vi "Add test result.vi"(10 "Test Result":T1, 11 "LUnit Test Case In":refnum<class "LUnit Test Case.lvclass">) -> (3 "LUnit Test Case Out":refnum<class "LUnit Test Case.lvclass">)   [LabVIEW 2020, in "LUnit Test Case.lvclass"]
uses:
  LUnit Test Case.lvclass
  Result Types/Assertion Result/Assertion Result.ctl
  Rewrite Project/Result/Status.ctl
  LUnit Test Case.lvclass/LUnit Test Case.ctl
  Result Types/Method Result/Public/Aggregate Assertion Results.vi
  Result Types/Method Result/Private/Merge Status.vi
  Result Types/Method Result/Private/Concatenate result strings.vi
  Result Types/Case Result/Test Case Result.lvlib
  Result Types/Assertion Result/Assertion Result.lvlib
  Rewrite Project/Result/Result.lvlib
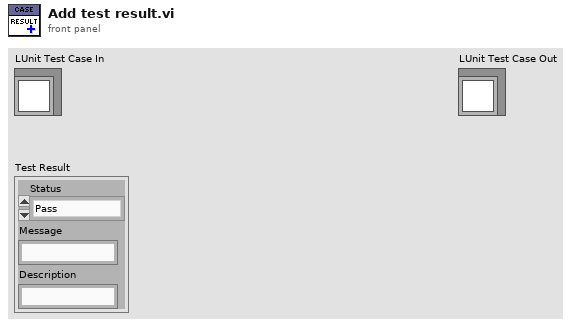
[diagram p1: front panel]
types:
  T1 = typedef "Assertion Result.lvlib/Assertion Result.ctl" = cluster{"Status":T2, "Message":string, "Description":string}
  T2 = typedef "Result.lvlib/Status.ctl" = enum16{"Pass", "Fail", "Error", "Skipped", "Setup Error", "Broken", "Teardown Error"}
  T3 = typedef "Test Case Result.lvlib/Test Case Result.ctl" = map{string, T4}
  T4 = typedef "Method Result.lvlib/Method Result.ctl" = cluster{"Test Case":string, "Test Method Name":string, "Status":T2, "Assertion Results":T1[], "Execution time":dbl, "Result String":string}
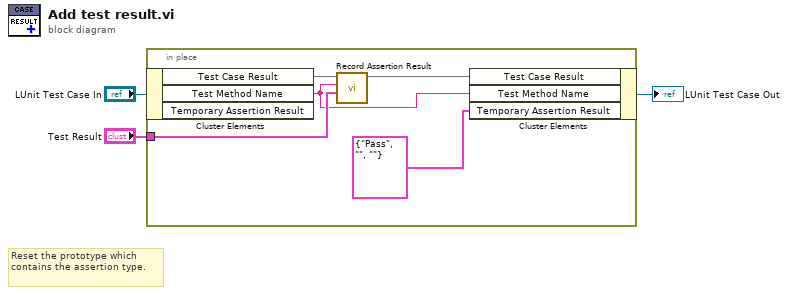
[diagram p0: block diagram]
diagram:
  # "Reset the prototype which contains the assertion type."
  n1 = in-place {
    in-place-border: "Test Result" -> [w8]
    n2 = in-place-cluster #1("LUnit Test Case In") -> ("Test Case Result"=w7:T3, "Test Method Name"=w5:string)  [unwired: 1 out]
    n3 = call "Record Assertion Result.vi"("Test Result"=w8, "Test Method"=w5, "Test Case Result in"=w7) -> ("Test Case Result out"=w6:T3)  [unwired: 8 in]
    n4 = in-place-cluster #1("Test Case Result"=w6, "Test Method Name"=w5, "Temporary Assertion Result"=T1 {"Status"=enum."Pass", "Message"="", "Description"=""}) -> (→"LUnit Test Case Out":refnum<class "LUnit Test Case.lvclass">)
  }
